vi "Get HP5385A Formated Parameters.vi"(8 "error in (no error)":errorcluster, 10 "Initial String":string, 11 "VISA Resource Name":refnum<visa-resource-name>) -> (0 "error out":errorcluster, 2 "Parameters":string, 3 "VISA Resource Name Out":refnum<visa-resource-name>, 4 "Data titles":string[](array[string])=["HP5385_Freque"])   [LabVIEW 2015]
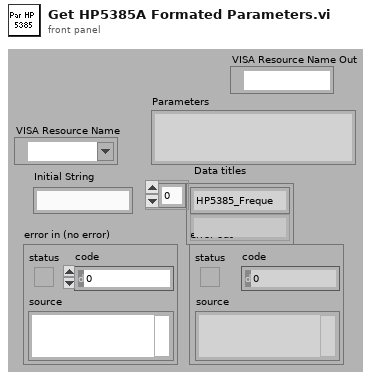
[diagram p1: front panel]
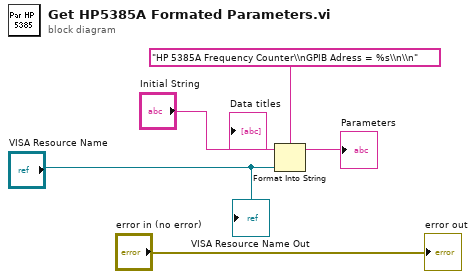
[diagram p0: block diagram]
diagram:
  n1 = Format Into String(format string="HP 5385A Frequency Counter\\nGPIB Adress = %s\\n\\n" ("string"), initial string="Initial String", "VISA Resource Name") -> (resulting string=→"Parameters":string)  [unwired: 1 in, 1 out]
  "error out" <- "error in (no error)"
  "VISA Resource Name Out" <- "VISA Resource Name"
